vi "状态机-3-红绿灯.vi"() -> ()   [LabVIEW 2023]
panel:
  out "Red":bool
  out "Yellow":bool
  in  "stop":bool
  out "Green":bool
  # "红绿灯"
  # "状态机 -3"
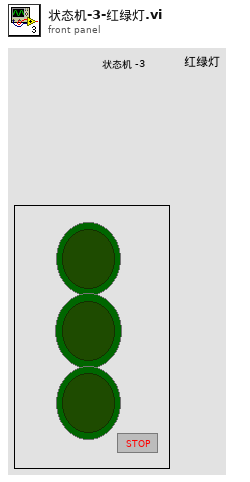
[diagram p1: front panel]
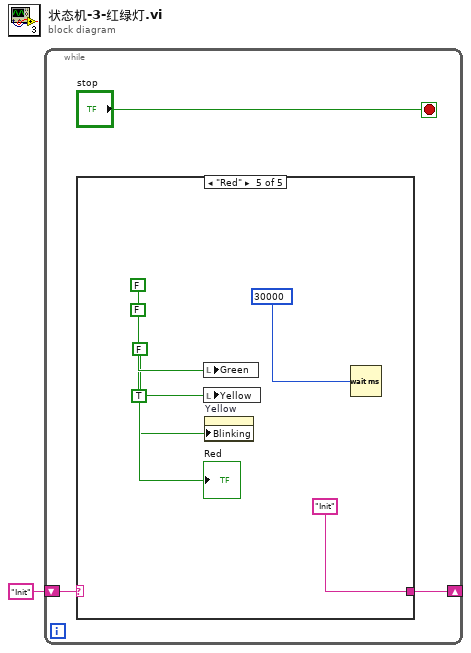
[diagram p0: block diagram]
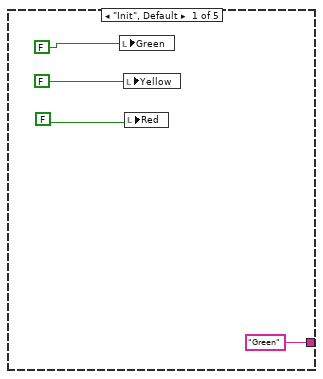
[diagram p2: hidden frame]
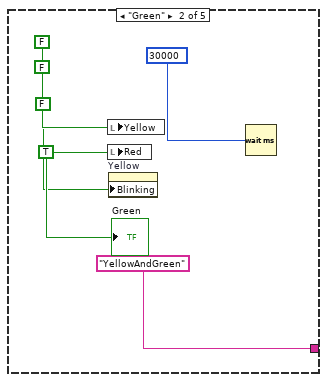
[diagram p3: hidden frame]
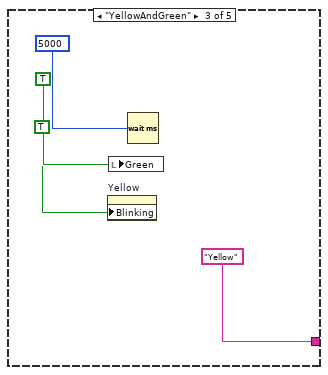
[diagram p4: hidden frame]
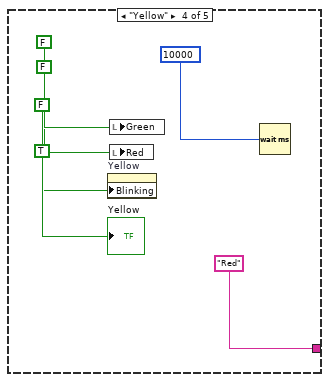
[diagram p5: hidden frame]
diagram:
  n1 = while {
    shift-right: [w3] -> _
    shift-left: "Init" -> [w4]
    stop <- "stop" stop-if-true
    n2 = case shown="\"Red\"" w4 {
      tunnel: ["Green" "YellowAndGreen" "Yellow" "Red" "Init"] -> w3
      frame "Init", Default {
        n3 = local write "Green"(FALSE) -> ()
        n4 = local write "Yellow"(FALSE) -> ()
        n5 = local write "Red"(FALSE) -> ()
      }
      frame "Green" {
        n6 = local write "Yellow"(FALSE) -> ()
        n7 = local write "Red"(FALSE ("Red")) -> ()
        n8 = property on="Yellow" class="Bool (strict)"("Blinking"=FALSE) -> ()  [unwired: 2 in, 2 out]
        n9 = Wait (ms)(milliseconds to wait=u32 30000) -> ()  [unwired: 1 out]
        "Green" <- TRUE ("Green")
      }
      frame "YellowAndGreen" {
        n10 = property on="Yellow" class="Bool (strict)"("Blinking"=TRUE) -> ()  [unwired: 2 in, 2 out]
        n11 = local write "Green"(TRUE) -> ()
        n12 = Wait (ms)(milliseconds to wait=u32 5000) -> ()  [unwired: 1 out]
      }
      frame "Yellow" {
        n13 = property on="Yellow" class="Bool (strict)"("Blinking"=FALSE) -> ()  [unwired: 2 in, 2 out]
        n14 = local write "Green"(FALSE) -> ()
        n15 = local write "Red"(FALSE ("Red")) -> ()
        n16 = Wait (ms)(milliseconds to wait=u32 10000) -> ()  [unwired: 1 out]
        "Yellow" <- TRUE ("Yellow")
      }
      frame "Red" {
        n17 = local write "Green"(FALSE ("Green")) -> ()
        n18 = local write "Yellow"(FALSE ("Yellow")) -> ()
        n19 = property on="Yellow" class="Bool (strict)"("Blinking"=FALSE) -> ()  [unwired: 2 in, 2 out]
        n20 = Wait (ms)(milliseconds to wait=u32 30000) -> ()  [unwired: 1 out]
        "Red" <- TRUE ("Red")
      }
    }
  }
